vi "LASER_SetAllIntensities.vi"(8 "error in":errorcluster, 11 "Intensitys":u8[](array[numeric])) -> (0 "error out":errorcluster)   [LabVIEW 2010]
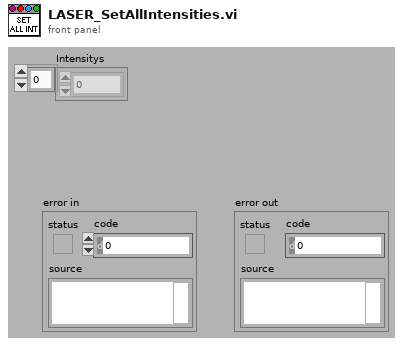
[diagram p1: front panel]
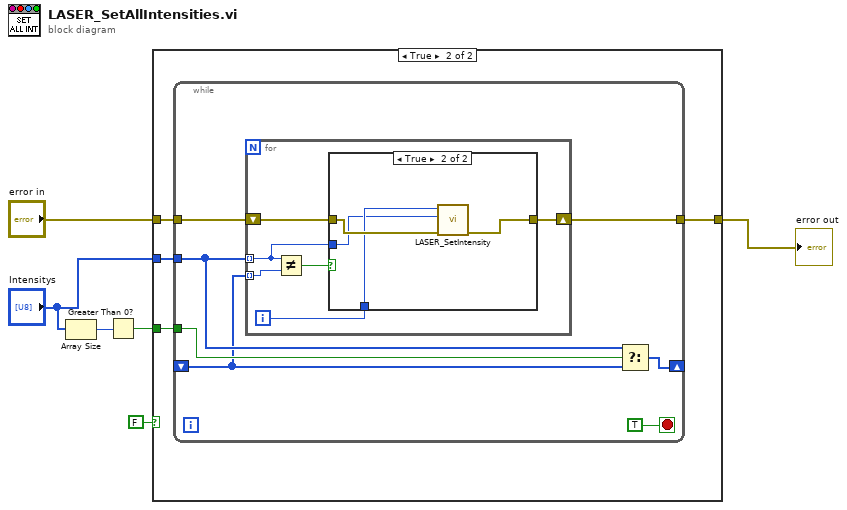
[diagram p0: block diagram]
diagram:
  n1 = Array Size(array="Intensitys") -> (size(s)=w2:i32)
  n2 = Greater Than 0?(x=w2) -> (x > 0?=w3:bool)
  n3 = case shown="True" FALSE {
    tunnel: [w7 w11] -> w6
    tunnel: "error in" -> [w7 w10]
    tunnel: "Intensitys" -> [_ w9]
    tunnel: w3 -> [_ w8]
    frame False {
    }
    frame True {
      n4 = while {
        tunnel: [w18] -> w11
        tunnel: w10 -> [w17]
        tunnel: w9 -> [w15]
        tunnel: w8 -> [w16]
        shift-right: [w14] -> _
        shift-left: _ -> [w13]
        stop <- TRUE stop-if-true
        n5 = for {
          tunnel: w13 -> [w24] mode=indexing
          tunnel: w15 -> [w19] mode=indexing
          shift-right: [w21] -> w18
          shift-left: w17 -> [w22]
          i -> [w20]
          n6 = Not Equal?(x=w19, y=w24) -> (x != y?=w23:bool)
          n7 = case shown="True" w23 {
            tunnel: w22 -> [w25 w29]
            tunnel: [w25 w28] -> w21
            tunnel: w20 -> [_ w27]
            tunnel: w19 -> [_ w26]
            frame False {
            }
            frame True {
              n8 = call "LASER_SetIntensity.vi"("error in"=w29, "Intensity"=w26, "LED Num"=w27) -> ("error out"=w28:errorcluster)  [unwired: 7 in]
            }
          }
        }
        n9 = Select(t=w15, s=w16, f=w13) -> (s? t:f=w14:u8[])
      }
    }
  }
  "error out" <- w6
